vi "Get 2D Time Stamp.vi"(7 "key description":string, 8 "sections":string[](array[string]), 9 "time stamp":timestamp[][](array[timestamp]), 11 "info data":string) -> (0 "sections out":string[](array[string]), 1 "key found?":bool, 2 "value":timestamp[][](array[timestamp]), 3 "info data out":string)   [LabVIEW 2020, in "infolib.lvlib"]
doc: "Reads matrix of time stamps. If section is entered it searches the key in the section(s).\nInput 'time stamp' can be used to set default value.\nIf key is not found, the output value is equal to 'time stamp' input.\nIf key is found, and some element of matrix cannot be converted into data type, the default value of output matrix element is based on:\n- first element of 'time stamp' input if available\n- otherwise date 01.01.1600T1:00:00 is used."
uses:
  infolib.lvlib
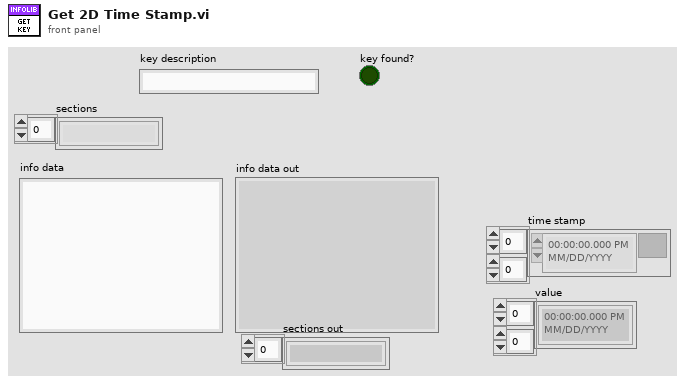
[diagram p1: front panel]
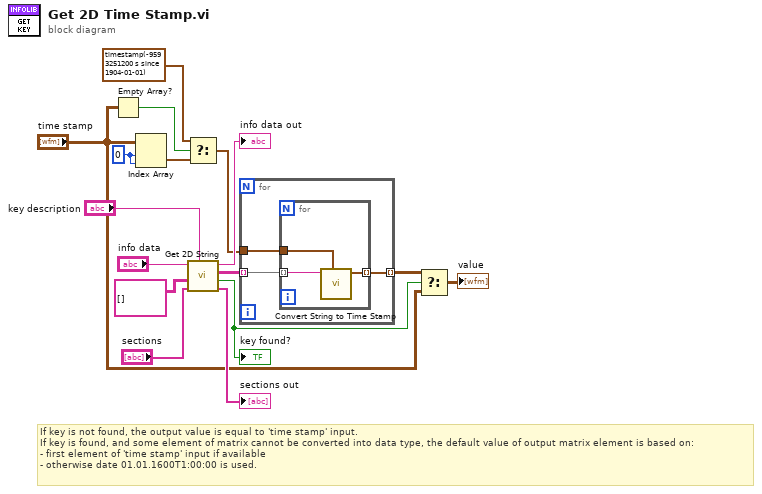
[diagram p0: block diagram]
diagram:
  w4 = 0 ("index (row)")
  # "If key is not found, the output value is equal to 'time stamp' input.\nIf key is found, and some element of matrix cannot be converted into data type, the default value of output matrix element is based on:\n- first element of 'time stamp' input if available\n- otherwise date 01.01.1600T1:00:00 is used."
  n1 = Empty Array?(array="time stamp") -> (empty?=w5:bool)
  n2 = Index Array(array="time stamp", index (row)=w4, index (col)=w4) -> (element=w6:timestamp)
  n3 = Select(t=timestamp(-9593251200 s since 1904-01-01) ("element"), s=w5, f=w6) -> (s? t:f=w2:timestamp)
  n4 = call "Get 2D String.vi"("key description"="key description", "sections"="sections", "string"=string[][] [] ("1D string array"), "info data"="info data") -> ("sections out"=→"sections out":string[], "key found?"=w9:bool, "value"=w10:string[][], "info data out"=→"info data out":string)  [unwired: 4 in]
  "key found?" <- w9
  n5 = for {
    tunnel: [w19] -> w8 mode=indexing
    tunnel: w10 -> [w18] mode=indexing
    tunnel: w2 -> [w17]
    n6 = for {
      tunnel: w18 -> [w22] mode=indexing
      tunnel: [w21] -> w19 mode=indexing
      tunnel: w17 -> [w20]
      n7 = call "Convert String to Time Stamp.vi"("default value of time stamp"=w20, "string"=w22) -> ("time stamp out"=w21:timestamp)  [unwired: 9 in]
    }
  }
  n8 = Select(t=w8, s=w9, f="time stamp") -> (s? t:f=→"value":timestamp[][])
